vi "Waveforms.Init.vi"(8 "error in":errorcluster, 11 "Channel.Paths":string[](array[string])) -> (0 "error out":errorcluster, 2 "WaveformStreaming.Event":refnum<event-registration>, 3 "Waveforms":T5)   [LabVIEW 2015, in "Station.Execution.lvlib"]
uses:
  <vilib>/NI Veristand/Execution/WaveformStreaming/Waveform Data Watcher Event Data (DBL).ctl
  <vilib>/NI Veristand/Execution/WaveformStreaming/WaveformStreamSpecification.ctl
  NationalInstruments.VeriStand.ClientAPI
  <vilib>/NI Veristand/Execution/WaveformStreaming/Registered Waveform Streams Data Event Refnum (DBL).ctl
  <vilib>/NI Veristand/Execution/WaveformStreaming/WaveformDataWatcherDBL.ctl
  <vilib>/NI Veristand/Execution/WaveformStreaming/WaveformStreamingAPI.ctl
  <vilib>/NI Veristand/Execution/WaveformStreaming/Set Rate for Waveform Stream (Acquisition Rate).vi
  <vilib>/NI Veristand/Execution/WaveformStreaming/Set Condition for Waveform Stream (All Data).vi
  <vilib>/NI Veristand/Execution/WaveformStreaming/Register for Waveform Data Events (DBL).vi
  Station.Execution.lvlib
  <vilib>/NI Veristand/Execution/WaveformStreaming/NI_VS Waveform Streaming Interface.lvlib
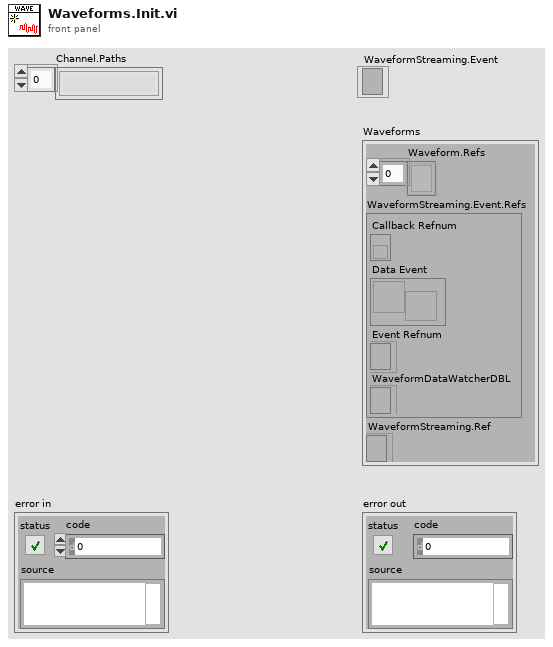
[diagram p1: front panel]
types:
  T1 = typedef "NI_VS Waveform Streaming Interface.lvlib/WaveformStreamSpecification.ctl" = refnum<k24>
  T2 = typedef "NI_VS Waveform Streaming Interface.lvlib/Registered Waveform Streams Data Event Refnum (DBL).ctl" = cluster{"Callback Refnum":refnum<k27>, "Data Event":refnum<user-event>, "Event Refnum":refnum<event-registration>, "WaveformDataWatcherDBL":T3}
  T3 = typedef "NI_VS Waveform Streaming Interface.lvlib/WaveformDataWatcherDBL.ctl" = refnum<k24>
  T4 = typedef "NI_VS Waveform Streaming Interface.lvlib/WaveformStreamingAPI.ctl" = refnum<k24>
  T5 = cluster{"Waveform.Refs":T1[], "WaveformStreaming.Event.Refs":T2, "WaveformStreaming.Ref":T4}
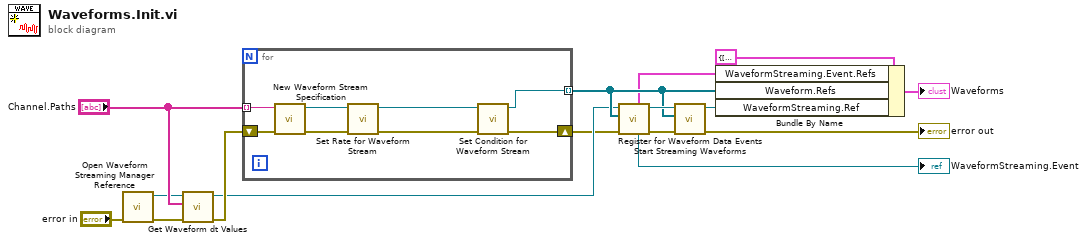
[diagram p0: block diagram]
diagram:
  n1 = call <vilib>:"Open Waveform Streaming Manager Reference.vi"("error in (no error)"="error in") -> ("error out"=w10:errorcluster, "WaveformStreaming"=w13:T4)  [unwired: 9 in]
  n2 = call <vilib>:"Get Waveform dt Values.vi"("error in (no error)"=w10, "waveform paths"="Channel.Paths", "WaveformStreaming in"=w13) -> ("error out"=w4:errorcluster, "WaveformStreaming out"=w2:T4)  [unwired: 6 in, 1 out]
  n3 = for {
    tunnel: "Channel.Paths" -> [w22] mode=indexing
    tunnel: [w19] -> w9 mode=indexing
    shift-right: [w18] -> w1
    shift-left: w4 -> [w17]
    n4 = call <vilib>:"New Waveform Stream Specification.vi"("error in (no error)"=w17, "waveform path"=w22) -> ("error out"=w24:errorcluster, "WaveformStreamSpecification"=w23:T1)  [unwired: 8 in]
    n5 = call-poly <vilib>:"Set Rate for Waveform Stream.vi"("error in (no error)"=w24, "WaveformStreamSpecification in"=w23) -> ("error out"=w21:errorcluster, "WaveformStreamSpecification out"=w20:T1)  [unwired: 8 in]
    n6 = call-poly <vilib>:"Set Condition for Waveform Stream.vi"("error in (no error)"=w21, "WaveformStreamSpecification in"=w20) -> ("error out"=w18:errorcluster, "WaveformStreamSpecification out"=w19:T1)  [unwired: 8 in]
  }
  n7 = call-poly <vilib>:"Register for Waveform Data Events.vi"("error in (no error)"=w1, "WaveformStreamSpecifications"=w9, "WaveformStreaming in"=w2) -> ("error out"=w11:errorcluster, "WaveformStreaming out"=w12:T4, "waveform data event registration (DBL)"=→"WaveformStreaming.Event":refnum<event-registration>, "registered waveform data event (DBL)"=w6:T2)  [unwired: 5 in]
  n8 = call <vilib>:"Start Streaming Waveforms.vi"("error in (no error)"=w11, "WaveformStreamSpecifications"=w9, "WaveformStreaming in"=w12) -> ("error out"=→"error out":errorcluster, "WaveformStreaming out"=w8:T4)  [unwired: 7 in]
  n9 = Bundle By Name(cluster=T5 {"Waveform.Refs"=[], "WaveformStreaming.Event.Refs"={"Callback Refnum"=refnum, "Data Event"=refnum, "Event Refnum"=refnum, "WaveformDataWatcherDBL"=refnum}, "WaveformStreaming.Ref"=refnum}, "WaveformStreaming.Event.Refs"=w6, "Waveform.Refs"=w9, "WaveformStreaming.Ref"=w8) -> (→"Waveforms":T5)
